vi "WRO_Bowling2.vi"() -> ()   [LabVIEW 2014]
doc: "The myRIO Project template acquires acceleration data from the onboard accelerometer and displays the changes of acceleration values in a waveform chart."
uses:
  <vilib>/vision/driver/NI_Vision_Acquisition_Software.lvlib
  <vilib>/vision/NI_Vision_Development_Module.lvlib
panel:
  out "장애물이니 다른 곳으로":bool=TRUE
  out "루프 횟수":i32
  in  "배경색밑 ROI 자름":dbl=5.0
  in  "Threshold Color Mode 3":enum32{"RGB", "HSL"}(radio)=enum."HSL"
  in  "Red or Hue 5":cluster{i32, i32}(slide)={0, 255} scale=0.0..255.0
  in  "Green or Saturation 5":cluster{i32, i32}(slide)={0, 35} scale=0.0..255.0
  in  "Blue or Luminance 5":cluster{i32, i32}(slide)={0, 65} scale=0.0..255.0
  out "볼링핀을찾았는가":bool=TRUE
  in  "화면전환":bool=TRUE
  out "Image 3":T1(plugin-control)
  in  "공 굴릴 범위":dbl=10.0
  in  "작게 움직이는 범위":dbl=60.0
  in  "탭컨트롤":dbl
  in  "탭 컨트롤":enum32{"볼링핀 0", "녹색핀 1"}(tab)
  in  "Blue or Luminance":cluster{i32, i32}(slide)={135, 255} scale=0.0..255.0
  in  "Green or Saturation":cluster{i32, i32}(slide)={0, 55} scale=0.0..255.0
  in  "Red or Hue":cluster{i32, i32}(slide)={0, 255} scale=0.0..255.0
  in  "Blue or Luminance 3":cluster{i32, i32}(slide)={60, 255} scale=0.0..255.0
  in  "Green or Saturation 3":cluster{i32, i32}(slide)={35, 255} scale=0.0..255.0
  in  "Red or Hue 3":cluster{i32, i32}(slide)={50, 130} scale=0.0..255.0
  out "초음파: 장애물?":bool
  out "초음파":dbl=321.76485464693883
  out "Acceleration 3":dbl(graph)=321.76485464693883
  in  "좌우모터":i16=25
  in  "Number of Erosion":i32=2
  in  "Threshold Color Mode":enum32{"RGB", "HSL"}(radio)=enum."HSL"
  out "Image 2":T1(plugin-control)
  out "Image":T1(plugin-control)
  in  "Camera Name":refnum<k21>="cam1" caption="IMAQdx Session"
  # "Control Motor"
  # "Read Encoder"
  # "초음파 거리"
  # "배경색(검은색) 색조"
  # "255"
  # "채도"
  # "HSL : 색조 채도 광도"
  # "35"
  # "광도"
  # "60"
  # "25"
  # "흰색 : 0/255"
  # "흰색 : 0~55"
  # "흰색 : 135~255"
  # "녹색 : 50/130"
  # "녹색 : 35/255"
  # "녹색 : 60/255"
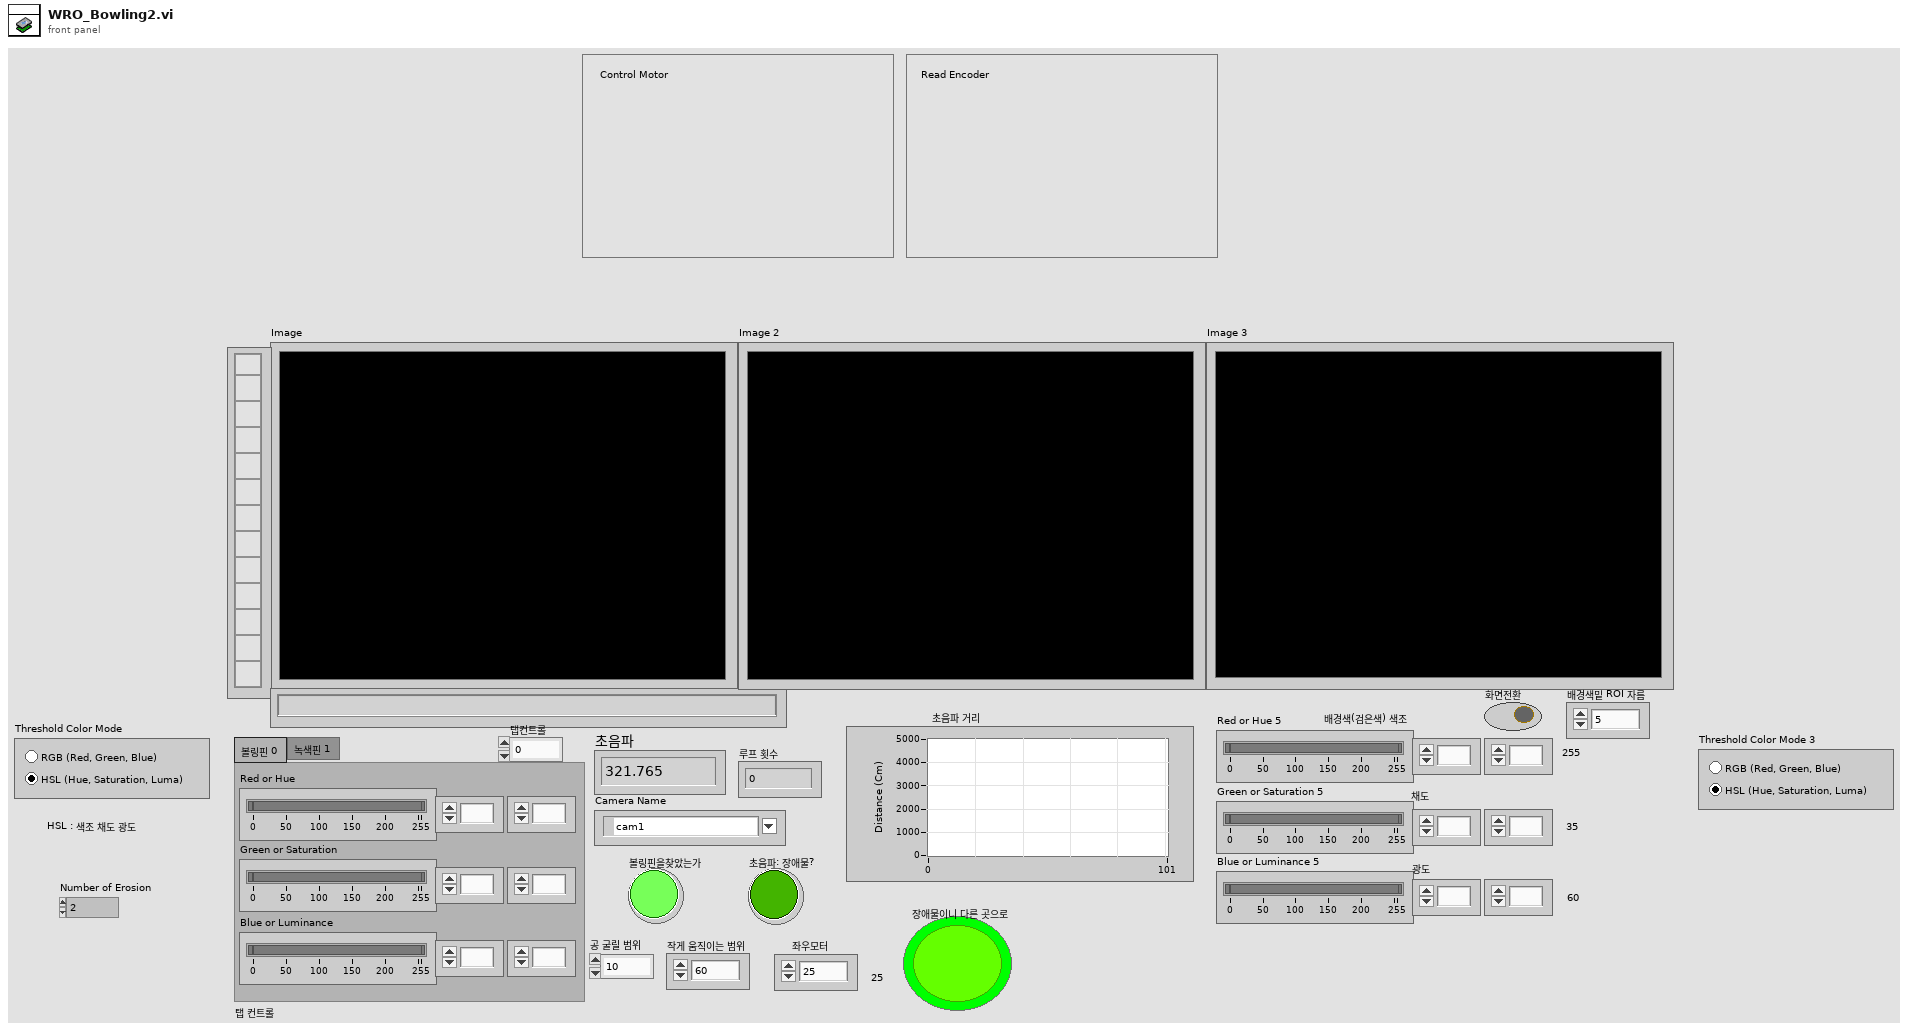
[diagram p1: front panel]
types:
  T1 = typedef "IMAQ Image.ctl" = refnum<image>
  T2 = typedef "IMAQ Rectangle" = cluster{"Left":i32, "Top":i32, "Right":i32, "Bottom":i32, "Rotation":dbl}
  T3 = typedef "Image Type" = u32
  T4 = typedef "IMAQdx.ctl" = refnum<k21>
  T5 = cluster{"Area":dbl, "Number of Holes":dbl, "Bounding Rect":cluster{"Left":dbl, "Top":dbl, "Right":dbl, "Bottom":dbl}, "Center of Mass":cluster{"X":dbl, "Y":dbl}, "Orientation":dbl, "Dimensions":cluster{"Width":dbl, "Height":dbl}}[]
  T6 = cluster{"Area":dbl, "Number of Holes":dbl, "Bounding Rect":cluster{"Left":dbl, "Top":dbl, "Right":dbl, "Bottom":dbl}, "Center of Mass":cluster{"X":dbl, "Y":dbl}, "Orientation":dbl, "Dimensions":cluster{"Width":dbl, "Height":dbl}}
  T7 = cluster{"Left":dbl, "Top":dbl, "Right":dbl, "Bottom":dbl}
  T8 = typedef "ROI Descriptor" = cluster{"Global Rectangle":i32[], "Contours":cluster{"ID":enum32{"External", "Internal"}, "Type":u32, "Coordinates":i32[]}[]}
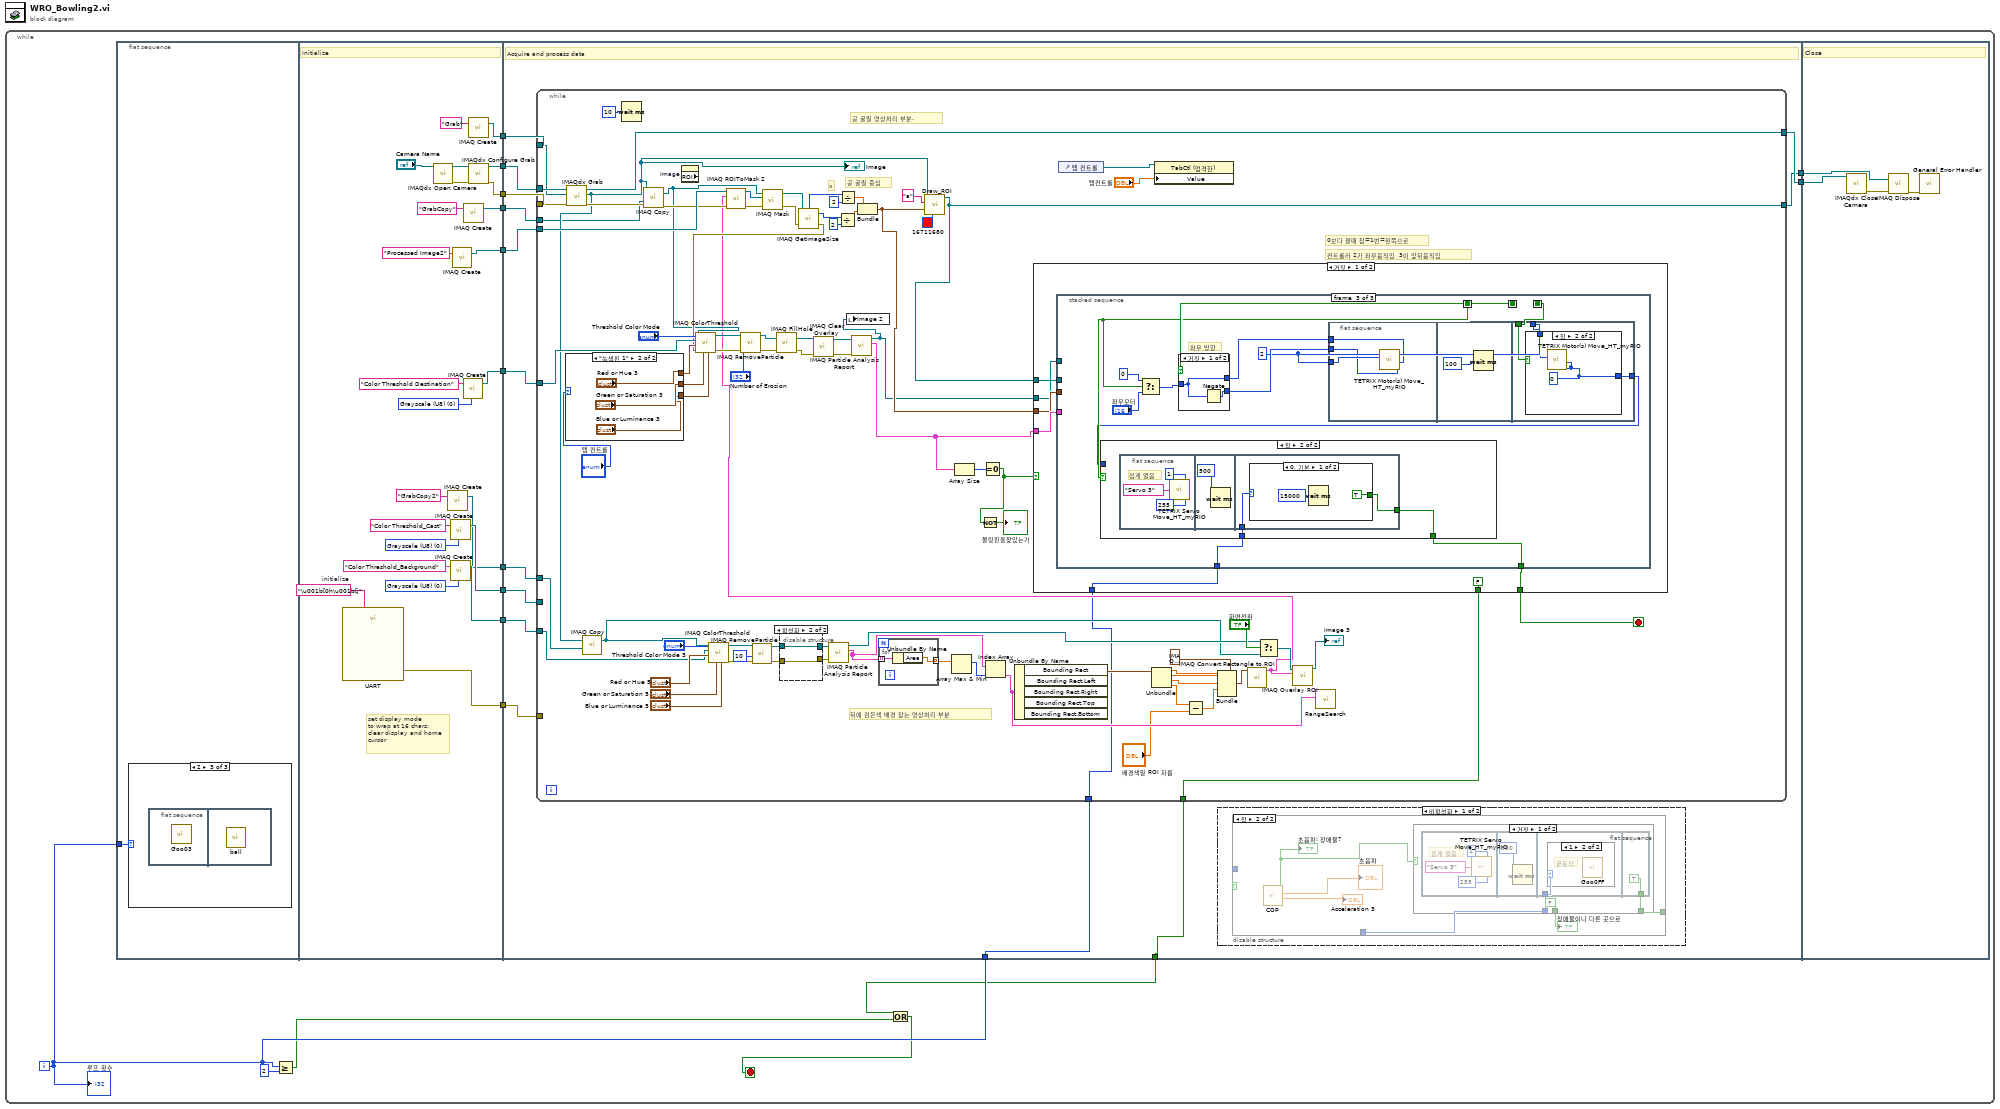
[diagram p0: block diagram]
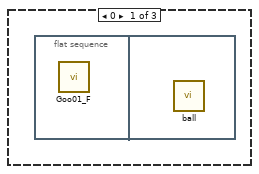
[diagram p2: hidden frame]
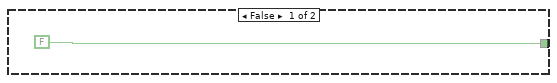
[diagram p4: hidden frame]
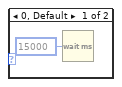
[diagram p5: hidden frame]
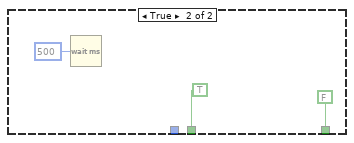
[diagram p6: hidden frame]
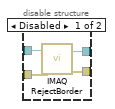
[diagram p8: hidden frame]
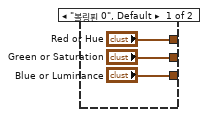
[diagram p9: hidden frame]
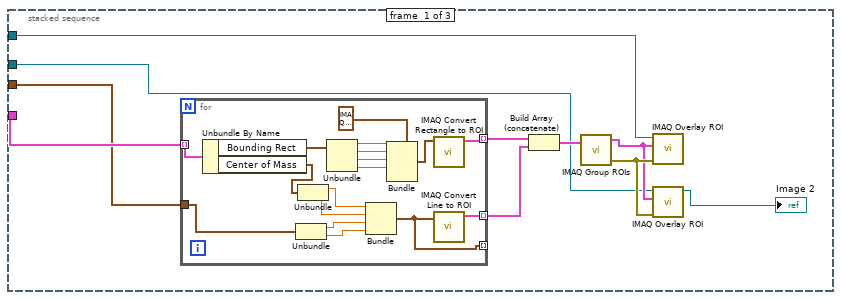
[diagram p10: hidden frame]
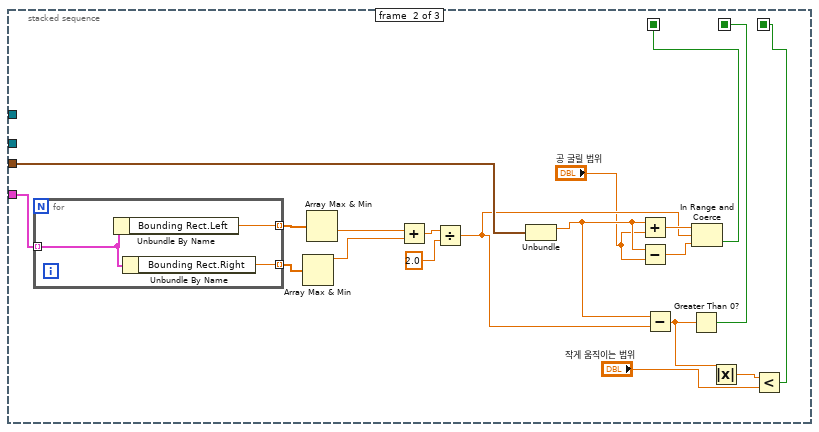
[diagram p11: hidden frame]
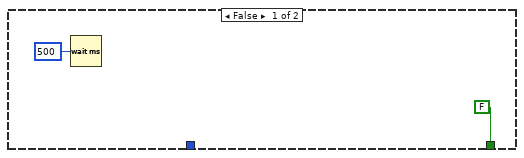
[diagram p12: hidden frame]
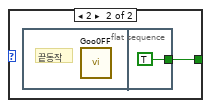
[diagram p13: hidden frame]
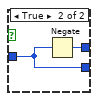
[diagram p15: hidden frame]
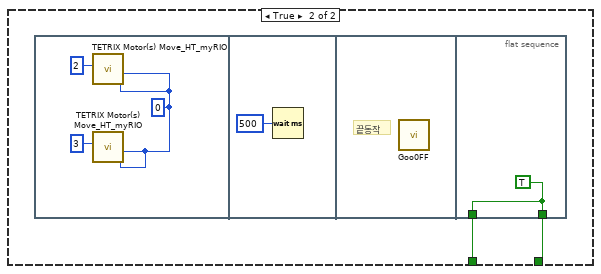
[diagram p16: hidden frame]
diagram:
  n1 = while {
    i -> [w4]
    stop <- w1 stop-if-true
    n2 = flat-sequence {
      tunnel: w4 -> [w18]
      tunnel: [w38] -> w17
      tunnel: [w37] -> w16
      tunnel: [w36] -> w15
      tunnel: [w34] -> w14
      tunnel: [w32] -> w13
      tunnel: [w31] -> w12
      tunnel: [w28] -> w11
      tunnel: [w24] -> w10
      tunnel: [w21] -> w9
      tunnel: [w19] -> w8
      tunnel: w17 -> [w56]
      tunnel: w16 -> [w55]
      tunnel: w15 -> [w54]
      tunnel: [w50] -> w7
      tunnel: [w53] -> w6
      tunnel: w14 -> [w52]
      tunnel: w13 -> [w51]
      tunnel: w12 -> [w44]
      tunnel: w11 -> [w49]
      tunnel: w10 -> [w48]
      tunnel: w9 -> [w47]
      tunnel: w8 -> [w46]
      tunnel: w4 -> [w45]
      tunnel: [w43] -> w3
      tunnel: w7 -> [w277]
      tunnel: w6 -> [w276]
      frame #0 {
        n3 = case shown="2" w18 {
          frame 0 {
            n4 = flat-sequence {
              frame #0 {
                n5 = call "Goo01_F.vi"() -> ()  [unwired: 12 in]
              }
              frame #1 {
                n6 = call "ball.vi"() -> ()  [unwired: 12 in]
              }
            }
          }
          frame 1, Default {
          }
          frame 2 {
            n7 = flat-sequence {
              frame #0 {
                n8 = call "Goo03.vi"() -> ()  [unwired: 12 in]
              }
              frame #1 {
                n9 = call "ball.vi"() -> ()  [unwired: 12 in]
              }
            }
          }
        }
      }
      frame #1 {
        w22 = T3 0 items=["Grayscale (U8)", "Grayscale (I16)", "Grayscale (SGL)", "Complex (CSG)", "RGB (U32)", "HSL (U32)", "RGB (U64)", "Grayscale (U16)"] ("Image Type")
        w25 = T3 0 items=["Grayscale (U8)", "Grayscale (I16)", "Grayscale (SGL)", "Complex (CSG)", "RGB (U32)", "HSL (U32)", "RGB (U64)", "Grayscale (U16)"] ("Image Type")
        w27 = "\u001b[0h\u001b[j"  # initialize
        w30 = T3 0 items=["Grayscale (U8)", "Grayscale (I16)", "Grayscale (SGL)", "Complex (CSG)", "RGB (U32)", "HSL (U32)", "RGB (U64)", "Grayscale (U16)"] ("Image Type")
        # "set display mode\nto wrap at 16 chars;\nclear display and home\ncursor"
        # "Initialize"
        n10 = call "UART"("Characters to Write"=w27) -> ("error out"=w31:errorcluster)  [unwired: 25 in, 1 out]
        n11 = call <vilib>:"IMAQdx Open Camera.vi"("Session In"="Camera Name") -> ("error out"=w42:errorcluster, "Session Out"=w41:T4)  [unwired: 2 in, 7 out]
        n12 = call "IMAQ Create"("Image Name"="GrabCopy2") -> ("New Image"=w19:T1)  [unwired: 3 in, 2 out]
        n13 = call "IMAQ Create"("Image Name"="Color Threshold_Cast", "Image Type"=w22) -> ("New Image"=w21:T1)  [unwired: 3 in, 1 out]
        n14 = call "IMAQ Create"("Image Name"="Color Threshold_Background", "Image Type"=w25) -> ("New Image"=w24:T1)  [unwired: 3 in, 1 out]
        n15 = call "IMAQ Create"("Image Name"="Processed Image2") -> ("New Image"=w34:T1)  [unwired: 3 in, 2 out]
        n16 = call "IMAQ Create"("Image Name"="Color Threshold Destination", "Image Type"=w30) -> ("New Image"=w28:T1)  [unwired: 3 in, 1 out]
        n17 = call "IMAQ Create"("Image Name"="GrabCopy") -> ("New Image"=w32:T1)  [unwired: 3 in, 2 out]
        n18 = call "IMAQ Create"("Image Name"="Grab") -> ("New Image"=w38:T1)  [unwired: 3 in, 2 out]
        n19 = call <vilib>:"IMAQdx Configure Grab.vi"("error in"=w42, "Session In"=w41) -> ("error out"=w36:errorcluster, "Session Out"=w37:T4)  [unwired: 8 out]
      }
      frame #2 {
        # "Acquire and process data"
        n20 = while {
          tunnel: [w156] -> w53
          tunnel: w54 -> [w158]
          tunnel: w55 -> [w159]
          tunnel: w56 -> [w157]
          tunnel: w52 -> [w154]
          tunnel: w51 -> [w85]
          tunnel: [w123] -> w50
          tunnel: w44 -> [_]
          tunnel: w49 -> [w141]
          tunnel: w48 -> [w96]
          tunnel: w47 -> [_]
          tunnel: w46 -> [w115]
          tunnel: w45 -> [w78]
          tunnel: [w77] -> w43
          stop <- w79 stop-if-true
          # "뒤에 검은색 배경 잡는 영상처리 부분"
          # "공 굴릴 영상처리 부분."
          # "0보다 클때 참=1번=왼쪽으로"
          # "컨트롤러 2가 좌우움직임  3이 앞뒤움직임"
          # "공 굴릴 중심"
          # "x"
          n21 = case shown="\"녹색핀 1\"" "탭 컨트롤" {
            tunnel: ["Blue or Luminance" "Blue or Luminance 3"] -> w139
            tunnel: ["Red or Hue" "Red or Hue 3"] -> w138
            tunnel: ["Green or Saturation" "Green or Saturation 3"] -> w137
            frame "볼링핀 0", Default {
            }
            frame "녹색핀 1" {
            }
          }
          n22 = call <vilib>:"IMAQdx Grab.vi"("error in"=w158, "Image In"=w157, "Session In"=w159) -> ("error out"=w144:errorcluster, "Image Out"=w86:T1, "Session Out"=w156:T4)  [unwired: 1 in, 5 out]
          "Image" <- w86
          n23 = call "IMAQ Copy"("Image Dst"=w115, "Image Src"=w86) -> ("Image Dst Out"=w92:T1)  [unwired: 4 in, 1 out]
          n24 = Wait (ms)(milliseconds to wait=u32 10 ("대기 시간(ms)")) -> ()  [unwired: 1 out]
          n25 = call "IMAQ Copy"("error in (no error)"=w144, "Image Dst"=w85, "Image Src"=w86) -> ("error out"=w143:errorcluster, "Image Dst Out"=w83:T1)  [unwired: 3 in]
          n26 = property on="Image" class="ImageControl" props=["ROI"]() -> ()  [unwired: 2 in, 3 out]
          n27 = call "IMAQ ColorThreshold"("Blue or Luma or Val or Inten Range"="Blue or Luminance 5", "Green or Sat Range"="Green or Saturation 5", "Color Mode"="Threshold Color Mode 3", "Red or Hue Range"="Red or Hue 5", "Image Dst"=w96, "Image Src"=w92) -> ("error out"=w103:errorcluster, "Image Dst Out"=w102:T1)  [unwired: 4 in]
          n28 = call "IMAQ RemoveParticle"("error in (no error)"=w103, "Number of Erosion"=10, "Image Src"=w102) -> ("error out"=w105:errorcluster, "Image Dst Out"=w104:T1)  [unwired: 7 in]
          n29 = disable-structure shown="활성화" {
            disable-tunnel: w104 -> [w163 w165]
            disable-tunnel: w105 -> [w162 w164]
            disable-tunnel: [w161 w165] -> w107
            disable-tunnel: [w160 w164] -> w108
            frame Disabled {
              n30 = call "IMAQ RejectBorder"("error in (no error)"=w162, "Image Src"=w163) -> ("error out"=w160:errorcluster, "Image Dst Out"=w161:T1)  [unwired: 4 in]
            }
            frame Enabled {
            }
          }
          n31 = call "IMAQ Particle Analysis Report"("error in (no error)"=w108, "Image"=w107) -> ("Particle Reports (Pixels)"=w98:T5, "Image Out (duplicate)"=w97:T1)  [unwired: 4 in, 4 out]
          n32 = for {
            tunnel: w98 -> [w167] mode=indexing
            tunnel: [w166] -> w121 mode=indexing
            n33 = Unbundle By Name(w167) -> ("Area"=w166:dbl)
          }
          n34 = Array Max & Min(array=w121) -> (max index (indices)=w120:i32)  [unwired: 3 out]
          n35 = Index Array(array=w98, index=w120) -> (element=w113:T6)
          n36 = Unbundle By Name(w113) -> ("Bounding Rect"=w117:T7)  [unwired: 4 out]
          n37 = control-ref of="탭 컨트롤"() -> (w127:refnum<vi>)
          n38 = Unbundle(w117) -> ("Left"=w95:dbl, "Top"=w118:dbl, "Right"=w94:dbl, "Bottom"=w91:dbl)
          n39 = property class="TabCtl (엄격한)"(reference=w127, "Value"="탭컨트롤") -> ()  [unwired: 1 in, 2 out]
          n40 = Subtract(x=w91, y="배경색밑 ROI 자름") -> (x-y=w90:dbl)
          n41 = Bundle(cluster=T2 {"Left"=0, "Top"=0, "Right"=0, "Bottom"=0, "Rotation"=0.0} ("Rectangle"), "Left"=w95, "Top"=w118, "Right"=w94, "Bottom"=w90) -> (w119:T2)  [unwired: 1 in]
          n42 = call "IMAQ Convert Rectangle to ROI"("Rectangle"=w119) -> ("ROI Descriptor"=w80:T8)  [unwired: 8 in, 1 out]
          n43 = call "IMAQ ROIToMask 2"("error in (no error)"=w143, "ROI Descriptor"=w80, "Image"=w154) -> ("error out"=w153:errorcluster, "Image Out"=w84:T1)  [unwired: 6 in, 1 out]
          n44 = call "IMAQ Mask"("error in (no error)"=w153, "Image Mask"=w84, "Image Src"=w83) -> ("error out"=w142:errorcluster, "Image Dst Out"=w87:T1)  [unwired: 2 in]
          n45 = call "IMAQ GetImageSize"("Image"=w87, "error in (no error)"=w142) -> ("Y Resolution"=w148:i32, "X Resolution"=w151:i32, "error out"=w134:errorcluster)  [unwired: 2 in]
          n46 = call "IMAQ ColorThreshold"("Blue or Luma or Val or Inten Range"=w139, "Green or Sat Range"=w137, "Color Mode"="Threshold Color Mode", "error in (no error)"=w134, "Red or Hue Range"=w138, "Image Dst"=w141, "Image Src"=w83) -> ("error out"=w135:errorcluster, "Image Dst Out"=w93:T1)  [unwired: 3 in]
          n47 = call "IMAQ RemoveParticle"("error in (no error)"=w135, "Number of Erosion"="Number of Erosion", "Image Src"=w93) -> ("error out"=w130:errorcluster, "Image Dst Out"=w131:T1)  [unwired: 7 in]
          n48 = call "IMAQ FillHole"("error in (no error)"=w130, "Image Src"=w131) -> ("error out"=w133:errorcluster, "Image Dst Out"=w132:T1)  [unwired: 4 in]
          n49 = call "IMAQ Clear Overlay"("error in (no error)"=w133, "Image"=w132) -> ("error out"=w152:errorcluster, "Image Out"=w155:T1)  [unwired: 1 in, 7 out]
          n50 = Divide(x=w148, y=2) -> (x/y=w147:dbl)
          n51 = Divide(x=w151, y=2) -> (x/y=w110:dbl)
          n52 = call "IMAQ Particle Analysis Report"("error in (no error)"=w152, "Image"=w155) -> ("Particle Reports (Pixels)"=w88:T5, "Image Out (duplicate)"=w122:T1)  [unwired: 4 in, 4 out]
          n53 = local write "Image 2"(w122) -> ()
          n54 = Bundle(w110, w147) -> (w125:cluster{dbl, dbl})  [unwired: 1 in]
          n55 = call "Draw_ROI.vi"("Color"=u32 16711680, "클러스터"=w125, "Group"="a", "참조 번호 입력"=w86) -> ("참조 번호 출력"=w123:T1)  [unwired: 7 in]
          n56 = Array Size(array=w88) -> (size(s)=w129:i32)
          n57 = Equal To 0?(x=w129) -> (x = 0?=w111:bool)
          n58 = Not(x=w111) -> (.not. x?=→"볼링핀을찾았는가":bool)
          n59 = case shown="거짓" w111 {
            tunnel: w88 -> [w180 _]
            tunnel: w125 -> [w179 _]
            tunnel: w122 -> [w178 _]
            tunnel: w123 -> [w177 _]
            tunnel: [w176 w270] -> w79
            tunnel: w78 -> [w174 _]
            tunnel: [FALSE w269] -> w77
            frame False {
              n60 = stacked-sequence {
                seq-local: [_ w208 _] -> [_ _ w239]
                seq-local: [_ w214 _] -> [_ _ w241]
                seq-local: [_ w210 _] -> [_ _ w240]
                tunnel: w180 -> [w185 w218 _]
                tunnel: w179 -> [w182 w217 _]
                tunnel: w178 -> [w184 _ _]
                tunnel: w177 -> [w183 _ _]
                tunnel: [_ _ w238] -> w176
                tunnel: w174 -> [_ _ w237]
                frame #0 {
                  n61 = for {
                    tunnel: w185 -> [w207] mode=indexing
                    tunnel: [w199] -> w187 mode=indexing
                    tunnel: w182 -> [w195]
                    tunnel: [w192] -> w189 mode=indexing
                    tunnel: [w191] -> _ mode=indexing
                    n62 = Unbundle By Name(w207) -> ("Bounding Rect"=w205:T7, "Center of Mass"=w198:cluster{"X":dbl, "Y":dbl})
                    n63 = Unbundle(w195) -> (w194:dbl, w193:dbl)
                    n64 = Unbundle(w198) -> ("X"=w197:dbl, "Y"=w196:dbl)
                    n65 = Unbundle(w205) -> ("Left"=w204:dbl, "Top"=w203:dbl, "Right"=w202:dbl, "Bottom"=w201:dbl)
                    n66 = Bundle("X"=w197, "Y"=w196, w194, w193) -> (w191:cluster{"X":dbl, "Y":dbl, dbl, dbl})  [unwired: 1 in]
                    n67 = Bundle(cluster=T2 {"Left"=0, "Top"=0, "Right"=0, "Bottom"=0, "Rotation"=0.0} ("Rectangle"), "Left"=w204, "Top"=w203, "Right"=w202, "Bottom"=w201) -> (w200:T2)  [unwired: 1 in]
                    n68 = call "IMAQ Convert Rectangle to ROI"("Rectangle"=w200) -> ("ROI Descriptor"=w199:T8)  [unwired: 8 in, 1 out]
                    n69 = call "IMAQ Convert Line to ROI"("Line"=w191) -> ("ROI Descriptor"=w192:T8)  [unwired: 8 in, 1 out]
                  }
                  n70 = Build Array (concatenate)(w187, w189) -> (w188:T8[])
                  n71 = call "IMAQ Group ROIs"("ROI Descriptors"=w188) -> ("error out"=w190:errorcluster, "ROI Descriptor out"=w186:T8)  [unwired: 1 in, 2 out]
                  n72 = call "IMAQ Overlay ROI"("error in (no error)"=w190, "ROI Descriptor"=w186, "Image"=w183) -> ()  [unwired: 3 in, 6 out]
                  n73 = call "IMAQ Overlay ROI"("error in (no error)"=w190, "ROI Descriptor"=w186, "Image"=w184) -> ("Image Out"=→"Image 2":T1)  [unwired: 3 in, 5 out]
                }
                frame #1 {
                  n74 = for {
                    tunnel: w218 -> [w229] mode=indexing
                    tunnel: [w228] -> w223 mode=indexing
                    tunnel: [w227] -> w225 mode=indexing
                    n75 = Unbundle By Name(w229) -> ("Bounding Rect.Left"=w228:dbl)
                    n76 = Unbundle By Name(w229) -> ("Bounding Rect.Right"=w227:dbl)
                  }
                  n77 = Array Max & Min(array=w225) -> (max value=w226:dbl)  [unwired: 3 out]
                  n78 = Array Max & Min(array=w223) -> (min value=w224:dbl)  [unwired: 3 out]
                  n79 = Add(x=w224, y=w226) -> (x+y=w219:dbl)
                  n80 = Divide(x=w219, y=2.0) -> (x/y=w215:dbl)
                  n81 = Unbundle(w217) -> (w216:dbl)  [unwired: 1 out]
                  n82 = Add(x=w216, y="공 굴릴 범위") -> (x+y=w221:dbl)
                  n83 = Subtract(x=w216, y="공 굴릴 범위") -> (x-y=w222:dbl)
                  n84 = Subtract(x=w216, y=w215) -> (x-y=w213:dbl)
                  n85 = Greater Than 0?(x=w213) -> (x > 0?=w214:bool)
                  n86 = In Range and Coerce(upper limit=w221, x=w215, lower limit=w222) -> (In Range?=w208:bool)  [unwired: 1 out]
                  n87 = Absolute Value(x=w213) -> (abs(x)=w212:dbl)
                  n88 = Less?(x=w212, y="작게 움직이는 범위") -> (x < y?=w210:bool)
                }
                frame #2 {
                  w232 = u8 2 ("Controller 2")
                  # "좌우 방향"
                  n89 = case shown="참" w239 {
                    tunnel: w230 -> [_ _]
                    tunnel: w237 -> [_ w245]
                    tunnel: [FALSE w244] -> w238
                    frame False {
                      n90 = Wait (ms)(milliseconds to wait=u32 500 ("대기 시간(ms)")) -> ()  [unwired: 1 out]
                    }
                    frame True {
                      n91 = flat-sequence {
                        tunnel: w245 -> [w251]
                        tunnel: [w250] -> w244
                        frame #0 {
                          # "집게 열음"
                          n92 = call <vilib>:"TETRIX Servo Move_HT_myRIO.vi"("Servo Position (0 - 255)"=u8 255, "Controller Daisy Chain Position (1 - 4)"=u8 1, "Select Servo"="Servo 3") -> ()  [unwired: 2 in, 1 out]
                        }
                        frame #1 {
                          n93 = Wait (ms)(milliseconds to wait=u32 500 ("대기 시간(ms)")) -> ()  [unwired: 1 out]
                        }
                        frame #2 {
                          n94 = case shown="0, 기본" w251 {
                            tunnel: [TRUE w254] -> w250
                            frame 0, Default {
                              n95 = Wait (ms)(milliseconds to wait=u32 15000 ("대기 시간(ms)")) -> ()  [unwired: 1 out]
                            }
                            frame 2 {
                              n96 = flat-sequence {
                                tunnel: [TRUE] -> w254
                                frame #0 {
                                # "끝동작"
                                n97 = call "Goo0FF.vi"() -> ()  [unwired: 12 in]
                                }
                                frame #1 {
                                }
                              }
                            }
                          }
                        }
                      }
                    }
                  }
                  n98 = Select(t=i8 0 ("Motor 2 Power (-100 to 100)\n0 = Stop/Brake\n-128 = Stop/Coast"), s=w239, f="좌우모터") -> (s? t:f=w234:i16)
                  n99 = case shown="거짓" w241 {
                    tunnel: [w266 w268] -> w236
                    tunnel: w234 -> [w266 w267]
                    tunnel: [w265 w267] -> w235
                    frame False {
                      n100 = Negate(x=w266) -> (-x=w265:i16)
                    }
                    frame True {
                      n101 = Negate(x=w267) -> (-x=w268:i16)
                    }
                  }
                  n102 = flat-sequence {
                    tunnel: w232 -> [w258]
                    tunnel: w236 -> [w257]
                    tunnel: w235 -> [w256]
                    tunnel: w232 -> [w262]
                    tunnel: w240 -> [w261]
                    tunnel: [w260] -> w230
                    frame #0 {
                      n103 = call <vilib>:"TETRIX Motor(s) Move_HT_myRIO.vi"("Motor 2 Power (-100 to 100)\n0 = Stop/Brake\n-128 = Stop/Coast"=w256, "Motor 1 Power (-100 to 100)\n0 = Stop/Brake\n-128 = Stop/Coast"=w257, "Controller Daisy Chain Position: 1 - 4"=w258) -> ()  [unwired: 6 in, 1 out]
                    }
                    frame #1 {
                      n104 = Wait (ms)(milliseconds to wait=u32 100 ("대기 시간(ms)")) -> ()  [unwired: 1 out]
                    }
                    frame #2 {
                      n105 = case shown="참" w261 {
                        tunnel: w262 -> [_ w264]
                        tunnel: [_ w263] -> w260
                        frame False {
                        }
                        frame True {
                          w263 = i8 0 ("Motor 2 Power (-100 to 100)\n0 = Stop/Brake\n-128 = Stop/Coast")
                          n106 = call <vilib>:"TETRIX Motor(s) Move_HT_myRIO.vi"("Motor 2 Power (-100 to 100)\n0 = Stop/Brake\n-128 = Stop/Coast"=w263, "Motor 1 Power (-100 to 100)\n0 = Stop/Brake\n-128 = Stop/Coast"=w263, "Controller Daisy Chain Position: 1 - 4"=w264) -> ()  [unwired: 6 in, 1 out]
                        }
                      }
                    }
                  }
                }
              }
            }
            frame True {
              n107 = flat-sequence {
                tunnel: [w275] -> w270
                tunnel: [w275] -> w269
                frame #0 {
                  w271 = 0
                  n108 = call <vilib>:"TETRIX Motor(s) Move_HT_myRIO.vi"("Motor 2 Power (-100 to 100)\n0 = Stop/Brake\n-128 = Stop/Coast"=w271, "Motor 1 Power (-100 to 100)\n0 = Stop/Brake\n-128 = Stop/Coast"=w271, "Controller Daisy Chain Position: 1 - 4"=u8 2) -> ()  [unwired: 6 in, 1 out]
                  n109 = call <vilib>:"TETRIX Motor(s) Move_HT_myRIO.vi"("Motor 2 Power (-100 to 100)\n0 = Stop/Brake\n-128 = Stop/Coast"=w271, "Motor 1 Power (-100 to 100)\n0 = Stop/Brake\n-128 = Stop/Coast"=w271, "Controller Daisy Chain Position: 1 - 4"=u8 3) -> ()  [unwired: 6 in, 1 out]
                }
                frame #1 {
                  n110 = Wait (ms)(milliseconds to wait=u32 500 ("대기 시간(ms)")) -> ()  [unwired: 1 out]
                }
                frame #2 {
                  # "끝동작"
                  n111 = call "Goo0FF.vi"() -> ()  [unwired: 12 in]
                }
                frame #3 {
                  w275 = TRUE
                }
              }
            }
          }
          n112 = Select(t=w97, s="화면전환", f=w92) -> (s? t:f=w82:T1)
          n113 = call "IMAQ Overlay ROI"("ROI Descriptor"=w80, "Image"=w82) -> ("Image Out"=→"Image 3":T1)  [unwired: 4 in, 5 out]
          n114 = call "RangeSearch.vi"("Particle Report"=w113) -> ()  [unwired: 10 in, 1 out]
        }
        n115 = disable-structure shown="비활성화" {
          frame Disabled {
            n116 = case shown="참" {
              selector: _ -> [_ _]
              tunnel: _ -> [_ _]
              tunnel: [FALSE w59] -> _
              tunnel: _ -> [_ w63]
              frame False {
              }
              frame True {
                n117 = call "COP.vi"() -> ("Acceleration 3"=→"Acceleration 3":dbl, "초음파"=→"초음파":dbl, "초음파: 장애물?"=w60:bool)  [unwired: 9 in]
                "초음파: 장애물?" <- w60
                n118 = case shown="거짓" w60 {
                  tunnel: w63 -> [w66 _]
                  tunnel: [w65 FALSE] -> w59
                  tunnel: [FALSE TRUE] -> w58
                  frame False {
                    n119 = flat-sequence {
                      tunnel: w66 -> [w71]
                      tunnel: [TRUE] -> w65
                      frame #0 {
                        # "집게 열음"
                        n120 = call <vilib>:"TETRIX Servo Move_HT_myRIO.vi"("Servo Position (0 - 255)"=u8 255, "Controller Daisy Chain Position (1 - 4)"=u8 1, "Select Servo"="Servo 3") -> ()  [unwired: 2 in, 1 out]
                      }
                      frame #1 {
                        n121 = Wait (ms)(milliseconds to wait=u32 500 ("대기 시간(ms)")) -> ()  [unwired: 1 out]
                      }
                      frame #2 {
                        n122 = case shown="1" w71 {
                          frame 0, Default {
                            n123 = Wait (ms)(milliseconds to wait=u32 15000 ("대기 시간(ms)")) -> ()  [unwired: 1 out]
                          }
                          frame 1 {
                            # "끝동작"
                            n124 = call "Goo0FF.vi"() -> ()  [unwired: 12 in]
                          }
                        }
                      }
                      frame #3 {
                      }
                    }
                  }
                  frame True {
                    n125 = Wait (ms)(milliseconds to wait=u32 500 ("대기 시간(ms)")) -> ()  [unwired: 1 out]
                  }
                }
                "장애물이니 다른 곳으로" <- w58
              }
            }
          }
          frame Enabled {
          }
        }
      }
      frame #3 {
        # "Close"
        n126 = call <vilib>:"IMAQdx Close Camera.vi"("Session In"=w276) -> ("error out"=w279:errorcluster)  [unwired: 1 in, 9 out]
        n127 = call "IMAQ Dispose"("Image"=w277, "error in (no error)"=w279) -> ("error out"=w278:errorcluster)  [unwired: 4 in]
        n128 = call <vilib>:"General Error Handler.vi"("error in (no error)"=w278) -> ()  [unwired: 2 in, 13 out]
      }
    }
    n129 = Greater Or Equal?(x=w4, y=2) -> (x >= y?=w2:bool)
    n130 = Or(x=w3, y=w2) -> (x .or. y?=w1:bool)
    "루프 횟수" <- w4
  }
